vi "ClsFlushInputBuffer.vi"(8 "error in (no error)":errorcluster, 11 "Connection In":u32) -> (0 "error out":errorcluster, 3 "Connection Out":u32)   [LabVIEW 2010]
doc: "Flush Input Buffer:\n\nFlush all the received data and command response, jump to the last valid position in the data stream from device.\n\nConnection In[Input]: the connection handle which is initially created by Open Connection subVI.\n\nConnection Out[Output]: the connection handle output which could be used for next subVI refering to the same connection.s"
uses:
  dependent dlls/CHRocodileDLL.dll
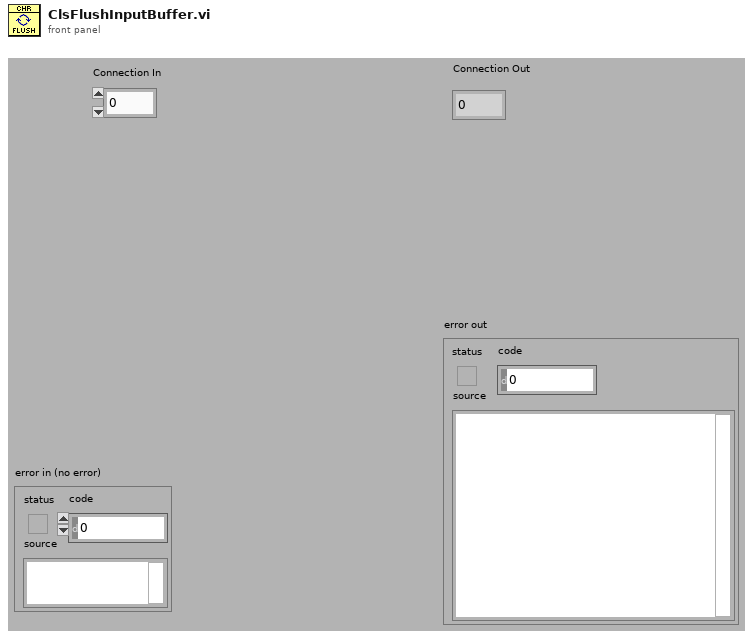
[diagram p1: front panel]
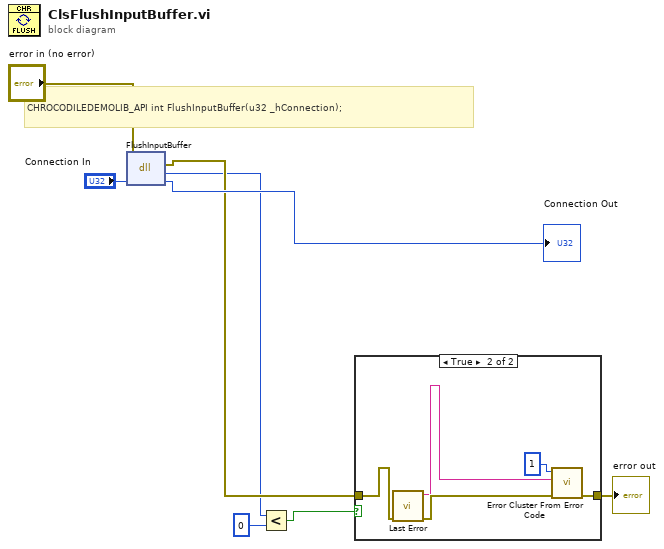
[diagram p0: block diagram]
diagram:
  # "CHROCODILEDEMOLIB_API int FlushInputBuffer(u32 _hConnection);"
  n1 = dll-call lib="C:/Users/y.ji/Documents/CHRocodile VIs/dependent dlls/CHRocodileDLL.dll" fn="FlushInputBuffer"(error in="error in (no error)", "_hConnection"="Connection In") -> (error out=w3:errorcluster, "return type"=w2:i32, "_hConnection"=→"Connection Out":u32)  [unwired: 2 in, 1 out]
  n2 = Less?(x=w2, y=0) -> (x < y?=w5:bool)
  n3 = case shown="True" w5 {
    tunnel: [w9 w13] -> w7
    tunnel: w3 -> [w9 w12]
    frame False {
    }
    frame True {
      n4 = call "Last Error.vi"("error in (no error)"=w12) -> ("error out"=w11:errorcluster, "Error Message"=w10:string)  [unwired: 9 in]
      n5 = call <vilib>:"Error Cluster From Error Code.vi"("error in (no error)"=w11, "error message (\"\")"=w10, "error code (0)"=1) -> ("error out"=w13:errorcluster)  [unwired: 6 in]
    }
  }
  "error out" <- w7
